vi "n平方和.vi"() -> ()   [LabVIEW 2015]
panel:
  out "平方和":string
  out "n的平方和":dbl
  in  "请输入n":dbl
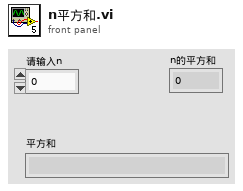
[diagram p1: front panel]
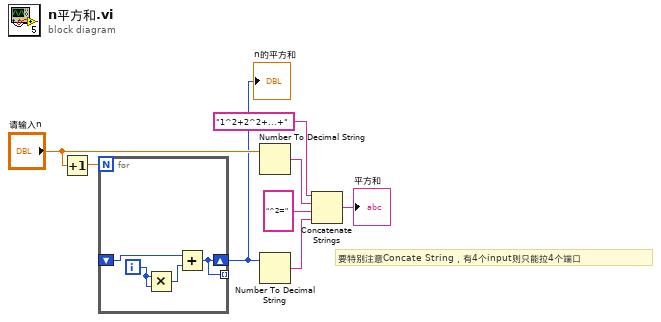
[diagram p0: block diagram]
diagram:
  # "要特别注意Concate String，有4个input则只能拉4个端口"
  n1 = Increment(x="请输入n") -> (x+1=w8:dbl)
  n2 = for {
    N: w8 -> [_]
    shift-right: [w9] -> w2
    shift-left: _ -> [w10]
    tunnel: [w9] -> _ mode=indexing
    i -> [w12]
    n3 = Multiply(x=w12, y=w12) -> (x*y=w11:i32)
    n4 = Add(x=w10, y=w11) -> (x+y=w9:i32)
  }
  "n的平方和" <- w2
  n5 = Number To Decimal String(number="请输入n") -> (decimal integer string=w3:string)  [unwired: 1 in]
  n6 = Number To Decimal String(number=w2) -> (decimal integer string=w1:string)  [unwired: 1 in]
  n7 = Concatenate Strings("1^2+2^2+...+", w3, "^2=", w1) -> (→"平方和":string)
